vi "AutonomousDrivePID.vi"(4 "ResetGyro":bool, 6 "ResetPosition":bool, 8 "error in (no error)":errorcluster, 9 "YSetpoint":dbl format="%.2f", 10 "XSetpoint":dbl format="%.2f", 11 "AngleSetpoint":dbl format="%.2f") -> ()   [LabVIEW 2014]
uses:
  Automated Tasks/AutomationGlobals.vi
  <vilib>/addons/control/pid/pid.llb/PID (DBL).vi
  <vilib>/addons/control/pid/NI_PID_pid.lvlib
panel:
  in  "Y PID gains":T1={"proportional gain (Kc)"=0.001, "integral time (Ti, min)"=0.0, "derivative time (Td, min)"=0.0} {"derivative time (Td, min)" format="%.3f"; "integral time (Ti, min)" format="%.3f"; "proportional gain (Kc)" format="%.3f"}
  in  "YRange":dbl=250.0
  in  "X PID gains":T1={"proportional gain (Kc)"=0.001, "integral time (Ti, min)"=0.0, "derivative time (Td, min)"=0.0} {"derivative time (Td, min)" format="%.3f"; "integral time (Ti, min)" format="%.3f"; "proportional gain (Kc)" format="%.3f"}
  in  "XRange":dbl=250.0
  out "Position Waveform Chart":dbl(graph)=1423.0
  in  "AngleRange":dbl=2.0
  out "Angle Waveform Chart":dbl(graph)=5.683606351592401
  in  "Angle PID gains":T1={"proportional gain (Kc)"=1.25, "integral time (Ti, min)"=0.0, "derivative time (Td, min)"=0.003} {"derivative time (Td, min)" format="%.3f"; "integral time (Ti, min)" format="%.3f"; "proportional gain (Kc)" format="%.3f"}
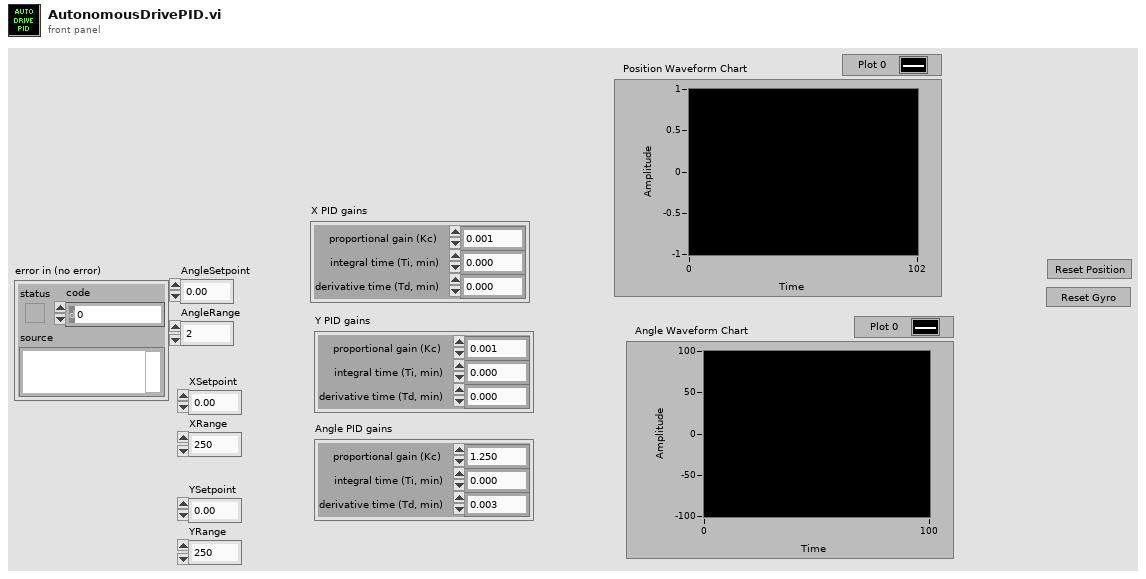
[diagram p1: front panel]
types:
  T1 = cluster{"proportional gain (Kc)":dbl, "integral time (Ti, min)":dbl, "derivative time (Td, min)":dbl}
  T2 = typedef "WPI_GyroDevRef.ctl" = cluster{"DevStatus":errorcluster, "Analog Module":T3, "Analog Channel":T4, "Offset":dbl, "Gain (VoltsPerDegree/Second)":dbl}
  T3 = typedef "FPGA_TypedefAnalogModule.ctl" = enum16{"Controller 1"}
  T4 = typedef "FPGA_AIChannel.ctl" = enum8{"AI 0", "AI 1", "AI 2", "AI 3", "AI MXP 0", "AI MXP 1", "AI MXP 2", "AI MXP 3", "Invalid"}
  T5 = typedef "WPI_MotorControlDeviceRef.ctl" = cluster{"DeviceStatus":errorcluster, "Type":T6, "PWM":cluster{"Controller":T7, "PWM Channel":T8, "DeadBand":T9}, "CAN":cluster{"Device Number":u8, "Control Mode":T10, "Semaphore":T11, "Max Vout":dbl, "TalonSRX Control Mode":T12}, "Invert":bool, "TransformRef":T13, "InvTransformRef":T13}
  T6 = typedef "WPI_MotorControlType.ctl" = enum16{"PWM", "CAN", "CANTalonSRX"}
  T7 = typedef "FPGA_TypedefDigitalModule.ctl" = enum16{"Controller 1"}
  T8 = typedef "FPGA_DIOPWMChannel.ctl" = enum8{"PWM 0", "PWM 1", "PWM 2", "PWM 3", "PWM 4", "PWM 5", "PWM 6", "PWM 7", "PWM 8", "PWM 9", "PWM MXP 0", "PWM MXP 1", "PWM MXP 2", "PWM MXP 3", "PWM MXP 4", "PWM MXP 5", "PWM MXP 6", "PWM MXP 7", "PWM MXP 8", "PWM MXP 9", "Invalid"}
  T9 = typedef "WPI_PWMDeadband.ctl" = cluster{"Name":string, "maxPositivePwm":i32, "minPositivePwm":i32, "centerPwm":i32, "maxNegativePwm":i32, "minNegativePwm":i32, "angularRange":u16}
  T10 = typedef "WPI_CANJaguar_ControlMode.ctl" = enum8{"Percent VBus", "Current", "Speed", "Position", "Voltage"}
  T11 = typedef "Semaphore RefNum" = refnum<k1>
  T12 = typedef "WPI_CANTalonSRX_APIControlMode.ctl" = enum8{"Percent VBus", "Speed", "Position", "Slave", "Unchanged / Invalid"}
  T13 = typedef "WPI_PWMTransform_ConPane.ctl" = refnum<vi>
  T14 = typedef "WPI_CANTalonSRX_GlobalStatus.ctl" = cluster{"Applied Throttle":dbl, "Module Enabled":bool, "CAN Error":errorcluster, "Closed Loop Error":dbl, "Forward Limit Switch Closed":bool, "Reverse Limit Switch Closed":bool, "Sensor Position":dbl, "Sensor Velocity":dbl, "Current":dbl, "Sticky Fault - Over Temp":bool, "Sticky Fault - Under Voltage":bool, "Sticky Fault - Forward Limit":bool, "Sticky Fault - Reverse Limit":bool, "Sticky Fault - Forward Soft Limit":bool, "Sticky Fault - Reverse Soft Limit":bool, "Brake is Enabled":bool, "Encoder Position":dbl, "Encoder Velocity":dbl, "Encoder Index Count":dbl, "Encoder A Pin State":bool, "Encoder B Pin State":bool, "Encoder Index Pin State":bool, "Analog In":dbl, "Analog In Velocity":dbl, "Temperature (C)":dbl, "Battery Voltage":dbl}
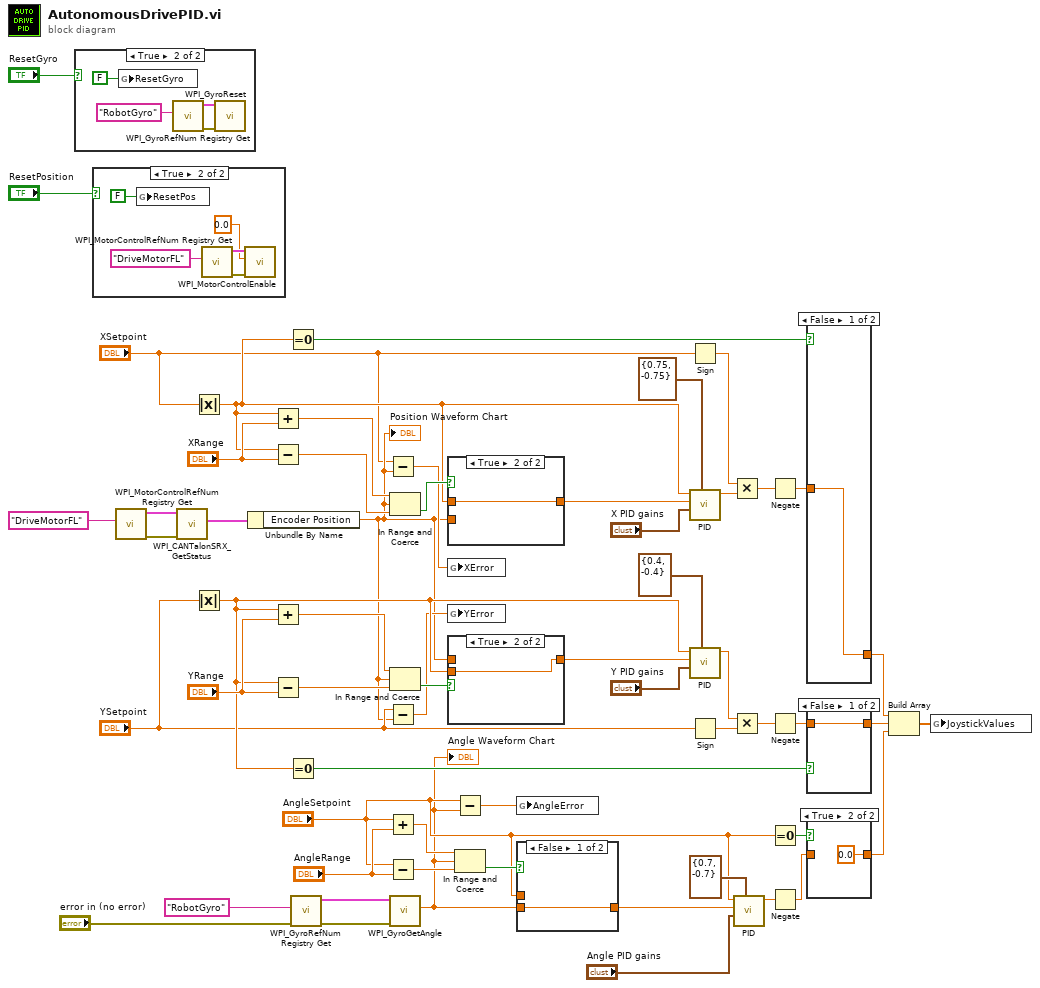
[diagram p0: block diagram]
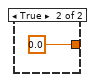
[diagram p5: hidden frame]
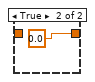
[diagram p6: hidden frame]
diagram:
  n1 = case shown="True" "ResetGyro" {
    frame False {
    }
    frame True {
      n2 = global write "AutomationGlobals.vi" "ResetGyro"(FALSE ("ResetGyro")) -> ()
      n3 = call <vilib>:"WPI_GyroRefNum Registry Get.vi"("refnum name"="RobotGyro") -> ("error out"=w61:errorcluster, "GyroDevRef"=w60:T2)  [unwired: 9 in]
      n4 = call <vilib>:"WPI_GyroReset.vi"("error in (no error)"=w61, "GyroDevRef"=w60) -> ()  [unwired: 8 in, 2 out]
    }
  }
  n5 = case shown="True" "ResetPosition" {
    frame False {
    }
    frame True {
      n6 = global write "AutomationGlobals.vi" "ResetPos"(FALSE ("ResetGyro")) -> ()
      n7 = call <vilib>:"WPI_MotorControlRefNum Registry Get.vi"("refnum name"="DriveMotorFL") -> ("error out"=w66:errorcluster, "MotorControlDevRef"=w65:T5)  [unwired: 9 in]
      n8 = call <vilib>:"WPI_MotorControlEnable.vi"("error in (no error)"=w66, "Encoder Initial Position"=0.0, "CAN Jaguar Ref"=w65) -> ()  [unwired: 7 in, 2 out]
    }
  }
  n9 = call <vilib>:"WPI_MotorControlRefNum Registry Get.vi"("refnum name"="DriveMotorFL") -> ("error out"=w45:errorcluster, "MotorControlDevRef"=w44:T5)  [unwired: 9 in]
  n10 = call <vilib>:"WPI_CANTalonSRX_GetStatus.vi"("error in (no error)"=w45, "CAN Talon SRX Ref"=w44) -> ("Talon SRX Status"=w43:T14)  [unwired: 7 in, 2 out]
  n11 = Absolute Value(x="XSetpoint") -> (abs(x)=w10:dbl)
  n12 = Absolute Value(x="YSetpoint") -> (abs(x)=w12:dbl)
  n13 = Unbundle By Name(w43) -> ("Encoder Position"=w5:dbl)
  "Position Waveform Chart" <- w5
  n14 = Add(x=w10, y="XRange") -> (x+y=w42:dbl)
  n15 = Subtract(x=w10, y="XRange") -> (x-y=w41:dbl)
  n16 = Add(x=w12, y="YRange") -> (x+y=w34:dbl)
  n17 = Subtract(x=w12, y="YRange") -> (x-y=w33:dbl)
  n18 = Equal To 0?(x=w10) -> (x = 0?=w20:bool)
  n19 = Equal To 0?(x=w12) -> (x = 0?=w19:bool)
  n20 = call <vilib>:"WPI_GyroRefNum Registry Get.vi"("error in (no error)"="error in (no error)", "refnum name"="RobotGyro") -> ("error out"=w57:errorcluster, "GyroDevRef"=w56:T2)  [unwired: 8 in]
  n21 = Subtract(x="XSetpoint", y=w5) -> (x-y=w6:dbl)
  n22 = Subtract(x="YSetpoint", y=w5) -> (x-y=w8:dbl)
  n23 = Add(x="AngleSetpoint", y="AngleRange") -> (x+y=w51:dbl)
  n24 = Subtract(x="AngleSetpoint", y="AngleRange") -> (x-y=w50:dbl)
  n25 = In Range and Coerce(upper limit=w42, x=w5, lower limit=w41) -> (In Range?=w39:bool)  [unwired: 1 out]
  n26 = In Range and Coerce(upper limit=w34, x=w5, lower limit=w33) -> (In Range?=w31:bool)  [unwired: 1 out]
  n27 = call <vilib>:"WPI_GyroGetAngle.vi"("error in (no error)"=w57, "GyroDevRef"=w56) -> ("Angle"=w1:dbl)  [unwired: 6 in, 3 out]
  "Angle Waveform Chart" <- w1
  n28 = case shown="True" w39 {
    tunnel: w10 -> [_ w69]
    tunnel: [w68 w69] -> w38
    tunnel: w5 -> [w68 _]
    frame False {
    }
    frame True {
    }
  }
  n29 = global write "AutomationGlobals.vi" "XError"(w6) -> ()
  n30 = global write "AutomationGlobals.vi" "YError"(w8) -> ()
  n31 = case shown="True" w31 {
    tunnel: w12 -> [_ w71]
    tunnel: [w70 w71] -> w30
    tunnel: w5 -> [w70 _]
    frame False {
    }
    frame True {
    }
  }
  n32 = Subtract(x="AngleSetpoint", y=w1) -> (x-y=w3:dbl)
  n33 = In Range and Coerce(upper limit=w51, x=w1, lower limit=w50) -> (In Range?=w49:bool)  [unwired: 1 out]
  n34 = global write "AutomationGlobals.vi" "AngleError"(w3) -> ()
  n35 = case shown="False" w49 {
    tunnel: "AngleSetpoint" -> [_ w73]
    tunnel: [w72 w73] -> w48
    tunnel: w1 -> [w72 _]
    frame False {
    }
    frame True {
    }
  }
  n36 = Sign(1:"XSetpoint") -> (0:w14:dbl)
  n37 = call-poly <vilib>:"PID.vi"("output range"=cluster{"output high":dbl, "output low":dbl} {"output high"=0.75, "output low"=-0.75}, "PID gains"="X PID gains", "process variable"=w38, "setpoint"=w10) -> ("output"=w35:dbl)  [unwired: 6 in, 1 out]
  n38 = call-poly <vilib>:"PID.vi"("output range"=cluster{"output high":dbl, "output low":dbl} {"output high"=0.4, "output low"=-0.4}, "PID gains"="Y PID gains", "process variable"=w30, "setpoint"=w12) -> ("output"=w24:dbl)  [unwired: 6 in, 1 out]
  n39 = Sign(1:"YSetpoint") -> (0:w11:dbl)
  n40 = Multiply(x=w14, y=w35) -> (x*y=w15:dbl)
  n41 = Multiply(x=w24, y=w11) -> (x*y=w13:dbl)
  n42 = call-poly <vilib>:"PID.vi"("output range"=cluster{"output high":dbl, "output low":dbl} {"output high"=0.7, "output low"=-0.7}, "PID gains"="Angle PID gains", "process variable"=w48, "setpoint"="AngleSetpoint") -> ("output"=w52:dbl)  [unwired: 6 in, 1 out]
  n43 = Negate(x=w15) -> (-x=w27:dbl)
  n44 = Negate(x=w13) -> (-x=w9:dbl)
  n45 = Equal To 0?(x="AngleSetpoint") -> (x = 0?=w18:bool)
  n46 = Negate(x=w52) -> (-x=w22:dbl)
  n47 = case shown="False" w20 {
    tunnel: w27 -> [w74 _]
    tunnel: [w74 0.0] -> w26
    frame False {
    }
    frame True {
    }
  }
  n48 = case shown="False" w19 {
    tunnel: [w76 0.0 ("output")] -> w25
    tunnel: w9 -> [w76 _]
    frame False {
    }
    frame True {
    }
  }
  n49 = case shown="True" w18 {
    tunnel: [w78 0.0] -> w23
    tunnel: w22 -> [w78 _]
    frame False {
    }
    frame True {
    }
  }
  n50 = Build Array(w26, w25, w23) -> (w21:dbl[])
  n51 = global write "AutomationGlobals.vi" "JoystickValues"(w21) -> ()
